vi "dfd_Validate MRate FXP for Code Gen.vi"(6 "output phase":i32, 7 "totalChan":i32=3, 8 "error in":errorcluster, 11 "multirate filter":T1={"mMRate_Structure"=enum."CIC", "mMRate_Mode"=0, "mMRate_Factor"=1, "mMRate_FIRParams"={"mMRate_FIR_H"=[], "mMRate_FIR_IsNyquist?"=FALSE, "mMRate_FIR_IsSymmetric?"=FALSE}, "mMRate_CICParams"={"mMRate_CIC_#Stage"=2, "mMRate_CIC_Lag"=1, "mMRate_CIC_Type"=enum."Lowpass"}, "mMRate_Order"=0, "mMRate_Version"="1.0", "mMRate_Comments"="", "mMRate_RationalFactor"={"mMRate_L"=-1, "mMRate_M"=-1}, "mMRate_Fs"=1.0, "mMRate_Quantized?"=FALSE, "mMRate_QFilterGain"=1.0, "mMRate_CoefWl"=16, "mMRate_Scaling"={"mMRate_ScaleByPowerOf2?"=FALSE, "mMRate_ScaleType"=enum."Time Domain 1-Norm"}, "mMRate_InputWl"=0, "mMRate_OutputWl"=0, "mMRate_OutputMode"=enum."Nearest", "mMRate_MultMode"=enum."Truncated", "mMRate_BitPruning"=FALSE, "mMRate_GainWl"=16, "mMRate_OutputFwl"=0, "mMRate_SumIwl"=0, "mMRate_InputIwl "=16, "mMRate_SumWl"=32, "mMRate_CoefIwl"=0} {"mMRate_SumWl" min=1 max=32 step=1; "mMRate_InputIwl" min=1 max=32 step=1; "mMRate_GainWl" min=1 max=32 step=1; "mMRate_OutputWl" min=1 max=32 step=1; "mMRate_InputWl" min=1 max=32 step=1; "mMRate_CoefWl" min=1 max=32 step=1; "mMRate_Mode" items=["Default"=-1, "No Rate Change"=0, "Interpolation"=1, "Decimation"=2, "Interpolated"=3, "Rational"=4]}) -> (0 "error out":errorcluster, 1 "memory cost":i32, 3 "multirate filter out":T1={"mMRate_Structure"=enum."CIC", "mMRate_Mode"=0, "mMRate_Factor"=1, "mMRate_FIRParams"={"mMRate_FIR_H"=[], "mMRate_FIR_IsNyquist?"=FALSE, "mMRate_FIR_IsSymmetric?"=FALSE}, "mMRate_CICParams"={"mMRate_CIC_#Stage"=2, "mMRate_CIC_Lag"=1, "mMRate_CIC_Type"=enum."Lowpass"}, "mMRate_Order"=0, "mMRate_Version"="1.0", "mMRate_Comments"="", "mMRate_RationalFactor"={"mMRate_L"=-1, "mMRate_M"=-1}, "mMRate_Fs"=1.0, "mMRate_Quantized?"=FALSE, "mMRate_QFilterGain"=1.0, "mMRate_CoefWl"=16, "mMRate_Scaling"={"mMRate_ScaleByPowerOf2?"=FALSE, "mMRate_ScaleType"=enum."Time Domain 1-Norm"}, "mMRate_InputWl"=0, "mMRate_OutputWl"=0, "mMRate_OutputMode"=enum."Nearest", "mMRate_MultMode"=enum."Truncated", "mMRate_BitPruning"=FALSE, "mMRate_GainWl"=16, "mMRate_OutputFwl"=0, "mMRate_SumIwl"=0, "mMRate_InputIwl "=16, "mMRate_SumWl"=32, "mMRate_CoefIwl"=0} {"mMRate_SumWl" min=1 max=32 step=1; "mMRate_InputIwl" min=1 max=32 step=1; "mMRate_GainWl" min=1 max=32 step=1; "mMRate_OutputWl" min=1 max=32 step=1; "mMRate_InputWl" min=1 max=32 step=1; "mMRate_CoefWl" min=1 max=32 step=1; "mMRate_Mode" items=["Default"=-1, "No Rate Change"=0, "Interpolation"=1, "Decimation"=2, "Interpolated"=3, "Rational"=4]})   [LabVIEW 2017, in "NI_DigFilterLicensed.lvlib"]
uses:
  <vilib>/addons/Digital Filter Design/NI_DigFilterLicensed.lvlib
  <vilib>/addons/Digital Filter Design/_Objects.llb/DFD Multirate Filter Obj.ctl
  <vilib>/addons/Digital Filter Design/_Objects.llb/DFD Multirate Mode.ctl
  <vilib>/addons/Digital Filter Design/_Objects.llb/DFD Coef Norm Type.ctl
  <vilib>/addons/Digital Filter Design/_Objects.llb/DFD Round-off Mode.ctl
  <vilib>/addons/Digital Filter Design/_Objects.llb/DFD FXP MRate Multiply Mode.ctl
  <vilib>/addons/Digital Filter Design/_Misc.llb/dfd_Error Handlers (Multiple).vi
  <vilib>/addons/Digital Filter Design/NI_DigFilter_FXP.lvlib
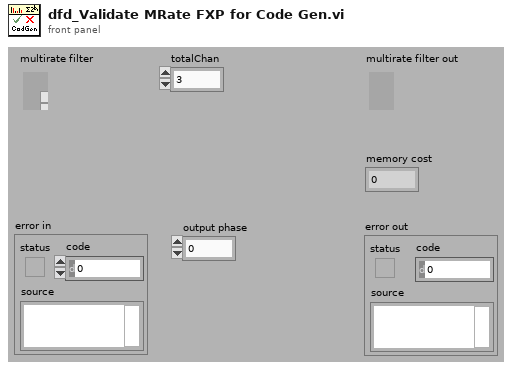
[diagram p1: front panel]
types:
  T1 = typedef "NI_DigFilterLicensed.lvlib/DFD Multirate Filter Obj.ctl" = cluster{"mMRate_Structure":enum16{"CIC", "FIR", "IIR", "Lattice"}, "mMRate_Mode":T2, "mMRate_Factor":i32, "mMRate_FIRParams":cluster{"mMRate_FIR_H":dbl[], "mMRate_FIR_IsNyquist?":bool, "mMRate_FIR_IsSymmetric?":bool}, "mMRate_CICParams":cluster{"mMRate_CIC_#Stage":i32, "mMRate_CIC_Lag":i32, "mMRate_CIC_Type":enum16{"Lowpass", "Highpass"}}, "mMRate_Order":i32, "mMRate_Version":string, "mMRate_Comments":string, "mMRate_RationalFactor":cluster{"mMRate_L":i32, "mMRate_M":i32}, "mMRate_Fs":dbl, "mMRate_Quantized?":bool, "mMRate_QFilterGain":dbl, "mMRate_CoefWl":i16, "mMRate_Scaling":cluster{"mMRate_ScaleByPowerOf2?":bool, "mMRate_ScaleType":T3}, "mMRate_InputWl":i16, "mMRate_OutputWl":i16, "mMRate_OutputMode":T4, "mMRate_MultMode":T5, "mMRate_BitPruning":bool, "mMRate_GainWl":i16, "mMRate_OutputFwl":i16, "mMRate_SumIwl":i16, "mMRate_InputIwl ":i16, "mMRate_SumWl":i16, "mMRate_CoefIwl":i16}
  T2 = typedef "NI_DigFilterLicensed.lvlib/DFD Multirate Mode.ctl" = i16
  T3 = typedef "NI_DigFilterLicensed.lvlib/DFD Coef Norm Type.ctl" = enum16{"No Norm", "Time Domain 1-Norm", "Time Domain 2-Norm", "Time Domain Inf-Norm"}
  T4 = typedef "NI_DigFilterLicensed.lvlib/DFD Round-off Mode.ctl" = enum16{"Nearest", "Truncation"}
  T5 = typedef "NI_DigFilterLicensed.lvlib/DFD FXP MRate Multiply Mode.ctl" = enum16{"Truncated", "Full"}
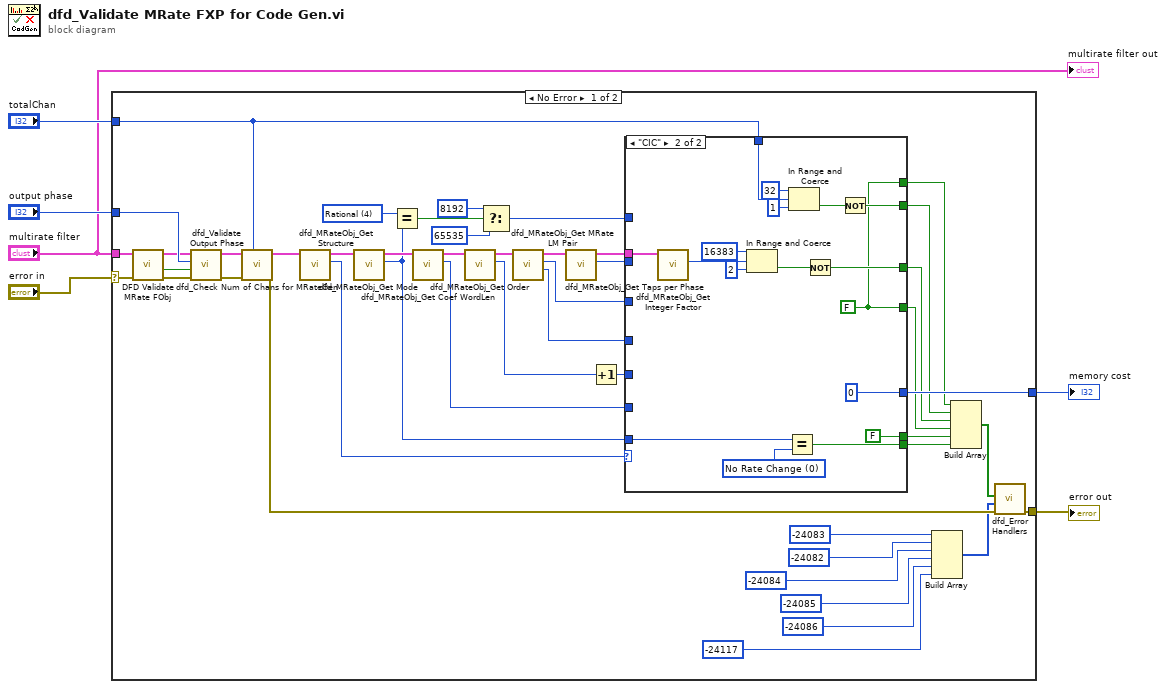
[diagram p0: block diagram]
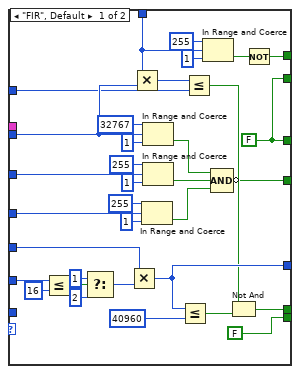
[diagram p2: hidden frame]
diagram:
  n1 = case shown="No Error" "error in" {
    selector: "error in" -> [w52 w104]
    tunnel: "multirate filter" -> [w14 _]
    tunnel: [w47 w104] -> w5
    tunnel: "output phase" -> [w51 _]
    tunnel: "totalChan" -> [w37 _]
    tunnel: [w45 _] -> w1
    frame No Error {
      w36 = T2 4 items=["Default"=-1, "No Rate Change"=0, "Interpolation"=1, "Decimation"=2, "Interpolated"=3, "Rational"=4] ("x")
      n2 = call <vilib>:"DFD Validate MRate FObj.vi"("error in (no error)"=w52, "multirate filter in"=w14) -> ("error out"=w44:errorcluster, "is valid FXP?"=w50:bool, "multirate filter out"=w43:T1)  [unwired: 7 out]
      n3 = call <vilib>:"dfd_Validate Output Phase.vi"("error in (no error)"=w44, "is valid FXP?"=w50, "output phase"=w51, "multirate filter in"=w43) -> ("error out"=w41:errorcluster, "dup multirate filter"=w42:T1)  [unwired: 6 out]
      n4 = call <vilib>:"dfd_Check Num of Chans for MRateGen.vi"("totalChan"=w37, "error in (no error)"=w41, "multirate filter"=w42) -> ("error out"=w39:errorcluster, "multirate filter out"=w40:T1)  [unwired: 7 out]
      n5 = call <vilib>:"dfd_MRateObj_Get Structure.vi"("multirate filter in"=w40) -> ("structure"=w48:enum16{"CIC", "FIR", "IIR", "Lattice"}, "dup multirate filter"=w49:T1)  [unwired: 9 out]
      n6 = call <vilib>:"dfd_MRateObj_Get Mode.vi"("multirate filter in"=w49) -> ("mode"=w13:T2, "dup multirate filter"=w31:T1)  [unwired: 9 out]
      n7 = Equal?(x=w36, y=w13) -> (x = y?=w35:bool)
      n8 = call <vilib>:"dfd_MRateObj_Get Coef WordLen.vi"("multirate filter in"=w31) -> ("coef wl"=w30:i16, "dup multirate filter"=w26:T1)  [unwired: 9 out]
      n9 = call <vilib>:"dfd_MRateObj_Get Order.vi"("multirate filter in"=w26) -> ("order"=w24:i32, "dup multirate filter"=w25:T1)  [unwired: 9 out]
      n10 = Select(t=8192, s=w35, f=65535 ("y")) -> (s? t:f=w32:i32)
      n11 = call <vilib>:"dfd_MRateObj_Get MRate LM Pair.vi"("multirate filter in"=w25) -> ("M"=w28:i32, "L"=w29:i32, "dup multirate filter"=w27:T1)  [unwired: 1 in, 7 out]
      n12 = call <vilib>:"dfd_MRateObj_Get Taps per Phase.vi"("multirate filter"=w27) -> ("taps per phase"=w38:i32, "multirate filter out"=w23:T1)  [unwired: 9 out]
      n13 = Increment(x=w24) -> (x+1=w46:i32)
      n14 = case shown="\"CIC\"" w48 {
        tunnel: w46 -> [w67 _]
        tunnel: w37 -> [w55 w92]
        tunnel: w29 -> [w69 _]
        tunnel: w28 -> [w86 _]
        tunnel: w30 -> [w85 _]
        tunnel: [w78 0] -> w45
        tunnel: w38 -> [w70 _]
        tunnel: w32 -> [w68 _]
        tunnel: w23 -> [_ w103]
        tunnel: [w64 FALSE] -> w22
        tunnel: [w60 w87] -> w21
        tunnel: [w58 w96] -> w20
        tunnel: w13 -> [_ w93]
        tunnel: [FALSE w94] -> w12
        tunnel: [w58 w88] -> w10
        tunnel: [w53 w87] -> w7
        frame "FIR", Default {
          w58 = FALSE
          n15 = Less Or Equal?(x=w85, y=i16 16) -> (x <= y?=w83:bool)
          n16 = Select(t=1, s=w83, f=2 ("t")) -> (s? t:f=w80:i32)
          n17 = Multiply(x=w67, y=w80) -> (x*y=w78:i32)
          n18 = Multiply(x=w55, y=w70) -> (x*y=w71:i32)
          n19 = In Range and Coerce(upper limit=255, x=w86, lower limit=1) -> (In Range?=w62:bool)  [unwired: 1 out]
          n20 = In Range and Coerce(upper limit=32767, x=w70, lower limit=1) -> (In Range?=w61:bool)  [unwired: 1 out]
          n21 = In Range and Coerce(upper limit=255, x=w69, lower limit=1) -> (In Range?=w63:bool)  [unwired: 1 out]
          n22 = Less Or Equal?(x=w78, y=40960) -> (x <= y?=w66:bool)
          n23 = Less Or Equal?(x=w71, y=w68) -> (x <= y?=w65:bool)
          n24 = In Range and Coerce(upper limit=255, x=w55, lower limit=1) -> (In Range?=w54:bool)  [unwired: 1 out]
          n25 = Compound Arithmetic op=AND(w61, w63, w62) -> (invert w60:bool)
          n26 = Not And(1:w66, 2:w65) -> (0:w64:bool)
          n27 = Not(x=w54) -> (.not. x?=w53:bool)
        }
        frame "CIC" {
          w95 = T2 0 items=["Default"=-1, "No Rate Change"=0, "Interpolation"=1, "Decimation"=2, "Interpolated"=3, "Rational"=4] ("mMRate_Mode")
          w87 = FALSE
          n28 = call <vilib>:"dfd_MRateObj_Get Integer Factor.vi"("multirate filter in"=w103) -> ("factor"=w100:i32)  [unwired: 10 out]
          n29 = In Range and Coerce(upper limit=16383, x=w100, lower limit=2) -> (In Range?=w97:bool)  [unwired: 1 out]
          n30 = Equal?(x=w93, y=w95) -> (x = y?=w94:bool)
          n31 = In Range and Coerce(upper limit=32, x=w92, lower limit=1) -> (In Range?=w89:bool)  [unwired: 1 out]
          n32 = Not(x=w97) -> (.not. x?=w96:bool)
          n33 = Not(x=w89) -> (.not. x?=w88:bool)
        }
      }
      n34 = Build Array(-24083 ("ERR_FIR_#CH"), -24082 ("ERR_CIC_#CH"), -24084 ("ERR_CIC_FACTOR_U16"), -24085 ("ERR_FIR_WL_U8"), -24086 ("ERR_MEM_FULL"), -24117 ("ERR_MA_CIC_NORATECHANGE")) -> (w15:i32[])
      n35 = Build Array(w7, w10, w20, w21, w22, w12) -> (w19:bool[])
      n36 = call-poly <vilib>:"dfd_Error Handlers.vi"("error in (no error)"=w39, "error sources"=w15, "condition failed?"=w19) -> ("error out"=w47:errorcluster)  [unwired: 8 out]
    }
    frame Error {
    }
  }
  "error out" <- w5
  "memory cost" <- w1
  "multirate filter out" <- "multirate filter"
